vi "LaunchProcess.vi"(8 "error in (no error)":errorcluster, 10 "Process Data":T1, 11 "JKI SMO in":refnum<class "JKI SMO.lvclass">) -> (0 "error out":errorcluster, 1 "VI Ref Out":refnum<vi>, 2 "Name":string, 3 "JKI SMO out":refnum<class "JKI SMO.lvclass">)   [LabVIEW 2013, in "JKI SMO.lvclass"]
doc: "Launches the Process VIs.\n\n---------------------------------------------------------------\nJKI State Machine Objects™\nhttp://jki.net/state-machine-objects/\nCopyright (C) 2005-2015, JKI <info@jki.net>\nALL RIGHTS RESERVED"
uses:
  JKI SMO.lvclass
  Typedefs/RegisteredProcessData--Cluster.ctl
panel:
  # "For instructions on how to use the JKI State Machine Objects, examples and video tutorials, visit:\nhttp://jki.net/state-machine-objects/\n\nJKI State Machine Objects™\nhttp://jki.net/state-machine-objects/\nCopyright (C) 2005-2015, JKI <info@jki.net>\nALL RIGHTS RESERVED"
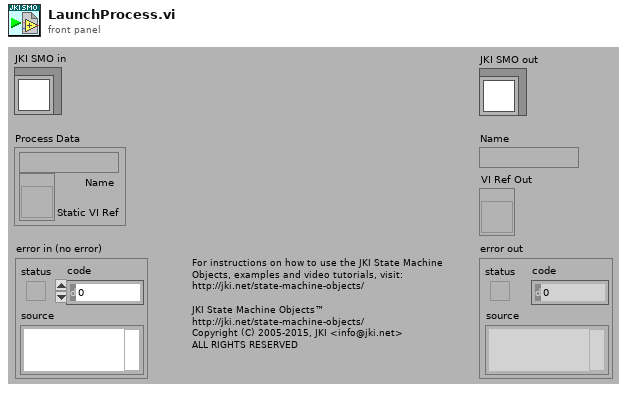
[diagram p1: front panel]
types:
  T1 = typedef "JKI SMO.lvclass/RegisteredProcessData--Cluster.ctl" = cluster{"Name":string, "Static VI Ref":refnum<vi>}
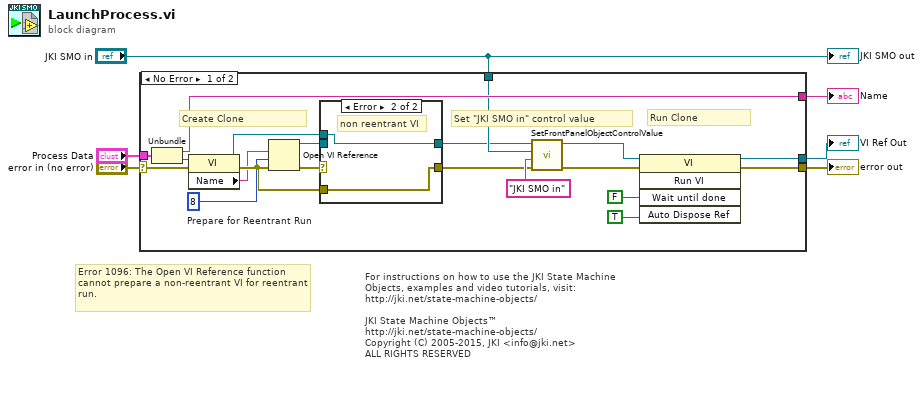
[diagram p0: block diagram]
diagram:
  # "For instructions on how to use the JKI State Machine Objects, examples and video tutorials, visit:\nhttp://jki.net/state-machine-objects/\n\nJKI State Machine Objects™\nhttp://jki.net/state-machine-objects/\nCopyright (C) 2005-2015, JKI <info@jki.net>\nALL RIGHTS RESERVED"
  # "Error 1096: The Open VI Reference function cannot prepare a non-reentrant VI for reentrant run."
  n1 = case shown="No Error" "error in (no error)" {
    selector: "error in (no error)" -> [w14 w31]
    tunnel: [w26 _] -> w6
    tunnel: "Process Data" -> [w24 _]
    tunnel: [w23 _] -> w4
    tunnel: [w20 w31] -> w3
    tunnel: "JKI SMO in" -> [w15 _]
    frame No Error {
      w19 = 8  # Prepare for Reentrant Run
      # "Run Clone"
      # "Set \"JKI SMO in\" control value"
      # "Create Clone"
      n2 = Unbundle(w24) -> ("Name"=w26:string, "Static VI Ref"=w25:refnum<vi>)
      n3 = property class="VI"(reference=w25, error in=w14) -> (reference out=w7:refnum<vi>, error out=w11:errorcluster, "Name"=w8:string)
      n4 = Open VI Reference(vi path=w8, options=w19, error in (no error)=w11) -> (vi reference=w10:refnum<vi>, error out=w13:errorcluster)  [unwired: 1 in, 2 out]
      n5 = case shown="Error" w13 {
        selector: w13 -> [w28 _]
        tunnel: [w28 w29] -> w12
        tunnel: w11 -> [_ w29]
        tunnel: w10 -> [w27 _]
        tunnel: [w27 w30] -> w9
        tunnel: w7 -> [_ w30]
        frame No Error {
        }
        frame Error {
          # "non reentrant VI"
        }
      }
      n6 = call "SetFrontPanelObjectControlValue.vi"("error in (no error)"=w12, "Control Name (\"\": Search by Type)"="JKI SMO in" ("Control Name (\"\": Search by Type)"), "JKI SMO in"=w15, "VI Ref In"=w9) -> ("error out"=w18:errorcluster, "VI Ref Out"=w22:refnum<vi>)  [unwired: 1 in, 5 out]
      n7 = invoke class="VI" method="Run VI"(reference=w22, error in=w18, "Wait until done"=FALSE ("Wait Until Done"), "Auto Dispose Ref"=TRUE ("Auto Dispose Reference")) -> (reference out=w23:refnum<vi>, error out=w20:errorcluster)  [unwired: 1 in, 3 out]
    }
    frame Error {
    }
  }
  "Name" <- w6
  "VI Ref Out" <- w4
  "error out" <- w3
  "JKI SMO out" <- "JKI SMO in"
